vi "ChannelPower.vi"(10 "MaxValue":dbl, 11 "AvgMaxValue":bool) -> (3 "Channel Power Cal":dbl)   [LabVIEW 2018]
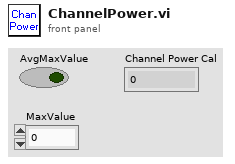
[diagram p1: front panel]
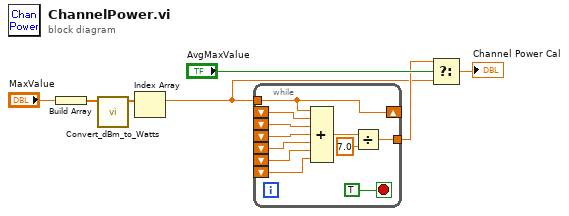
[diagram p0: block diagram]
diagram:
  n1 = Build Array("MaxValue") -> (w3:dbl[])
  n2 = call "Convert_dBm_to_Watts.vi"("P(dBm)"=w3) -> ("P(n_watts)"=w4:dbl[])  [unwired: 10 in]
  n3 = Index Array(array=w4) -> (element=w2:dbl)  [unwired: 1 in]
  n4 = while {
    shift-right: [w8] -> _
    shift-left: _ -> [w18]
    shift-left: _ -> [w17]
    shift-left: _ -> [w14]
    shift-left: _ -> [w13]
    shift-left: _ -> [w12]
    shift-left: _ -> [w11]
    tunnel: [w10] -> w6
    tunnel: w2 -> [w8]
    stop <- TRUE stop-if-true
    n5 = Compound Arithmetic op=ADD(w8, w18, w17, w14, w13, w12, w11) -> (w16:dbl)
    n6 = Divide(x=w16, y=7.0) -> (x/y=w10:dbl)
  }
  n7 = Select(t=w6, s="AvgMaxValue", f=w2) -> (s? t:f=→"Channel Power Cal":dbl)
